vi "AixplorerArbitraryLoad.vi"() -> ()   [LabVIEW 2015]
uses:
  Tek shared libraries/ArbitraryFunctions/VImode.vi
  General Libraries/Sequences.lvlib
  Tek shared libraries/ArbitraryFunctions.lvlib
  Read and Save Files/RW_Protocols.lvlib
panel:
  in  "CH2":bool
  in  "CH1":bool
  in  "event trig":bool
  in  "run":bool
  in  "WaveDuration (us)":dbl=2e-05
  out "sample rate (Hz) 2":dbl
  in  "Freq US (Hz)":dbl=6000000.0
  in  "?":T1(tab)
  in  "Sequence Loop Initialization":T2(array[cluster])=[{"min"=0.0, "step"=0.25, "max"=1.0, "name"="Phase"}, {"min"=1.0, "step"=1.0, "max"=3.0, "name"="Harmonic"}]
  in  "manual sequence":bool
  in  "load data log":bool
  in  "Multicolumn Listbox":i32[](listbox)
  out "Waveform Graph":dbl[][](graph)
  in  "FileName":string="LogFile.csv"
  in  "Enum":enum16{"sinus", "triangle"}(ring)=enum."triangle"
  in  "N average":i32=500
  out "Freq CH2 (Hz)":dbl=100000.0
  in  "clear waveforms":bool
  in  "define waveform CH1":bool
  out "Low Frequency OUT":dbl=100000.0
  out "High Frequency OUT":dbl=100000.0
  out "error out":errorcluster
  in  "load sequence CH1":bool
  in  "channel":enum16{"CH1", "CH2"}(ring)=enum."CH2"
  in  "CH1 (VOLT)":dbl=0.5
  out "capabilities":T3
  in  "sequence repeat":i32=500
  in  "sample rate (Hz)":dbl
  in  "define waveform CH 2":bool
  in  "other button":bool
  in  "Stop Button":bool
  in  "resource name":refnum<k15>
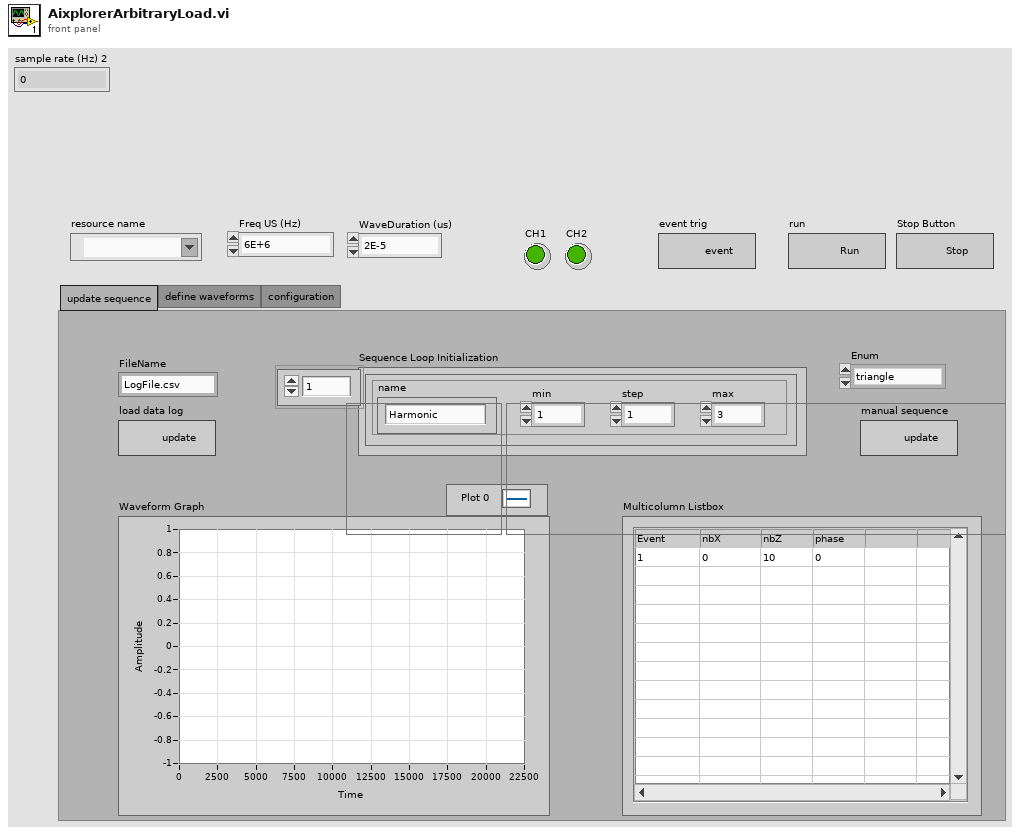
[diagram p1: front panel]
types:
  T1 = enum32{"update sequence", "define waveforms", "configuration"}
  T2 = cluster{"min":dbl, "step":dbl, "max":dbl, "name":string}[]
  T3 = cluster{"Max Number Of Sequences":i32, "Min Sequence Length":i32, "Max Sequence Length":i32, "Max Loop Count":i32}
  T4 = enum8{"Enabled", "Disabled", "Disabled and Grayed Out"}
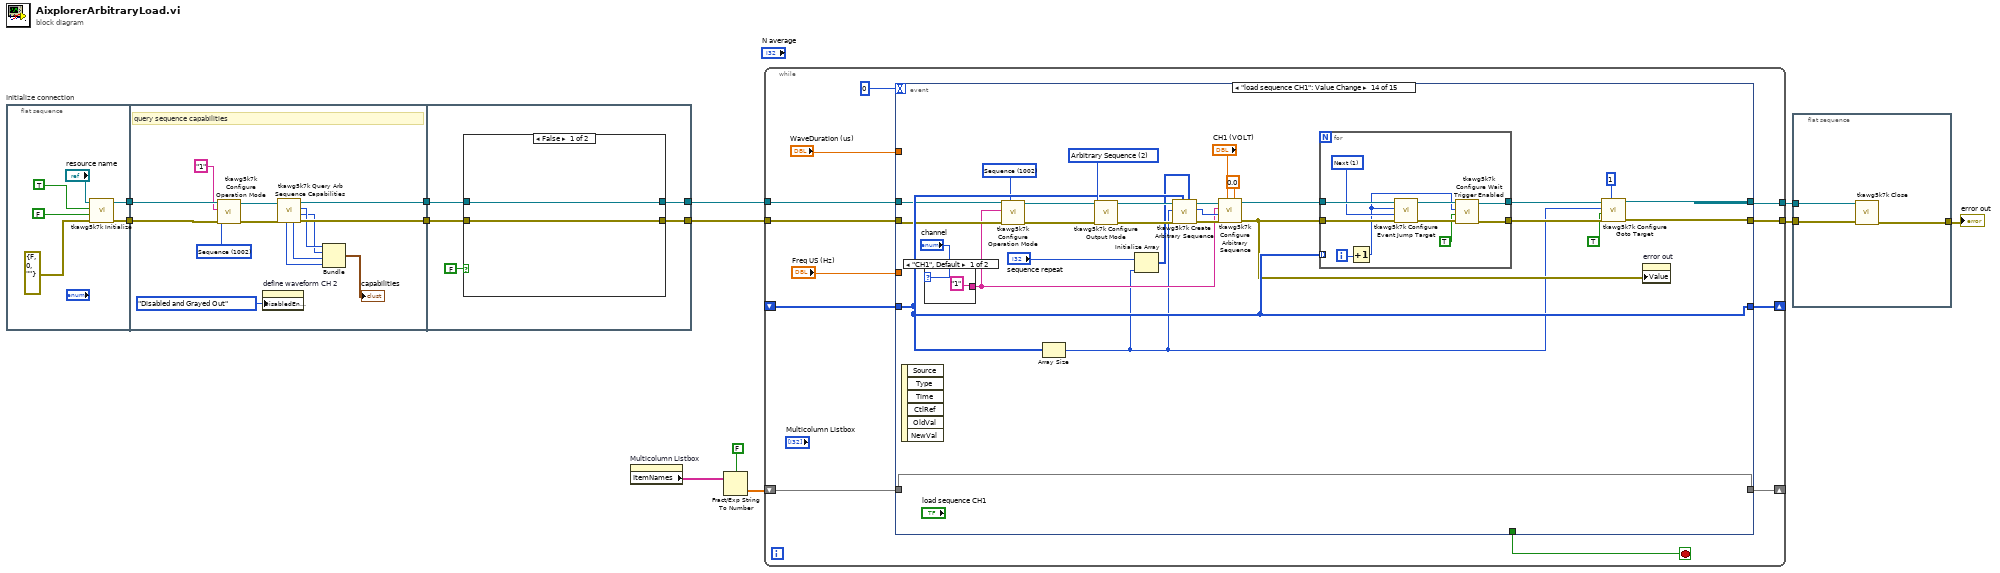
[diagram p0: block diagram]
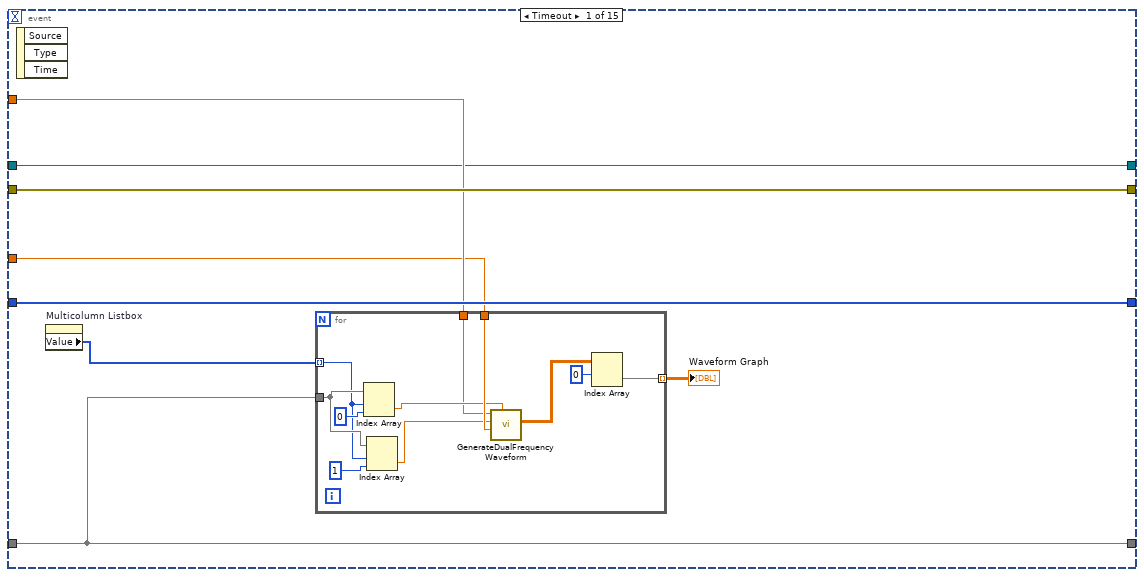
[diagram p2: hidden frame]
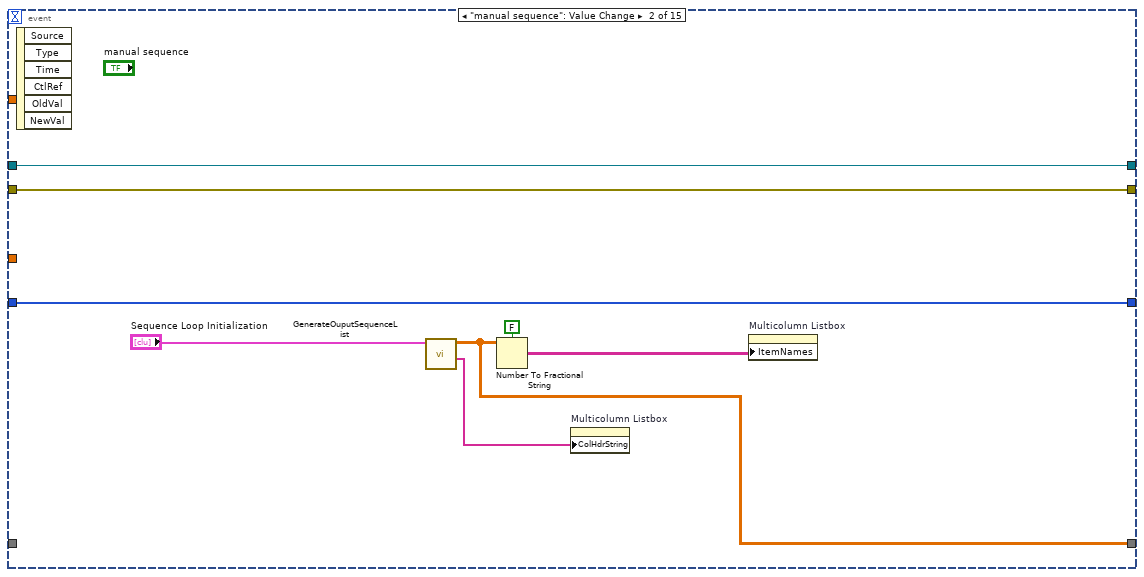
[diagram p3: hidden frame]
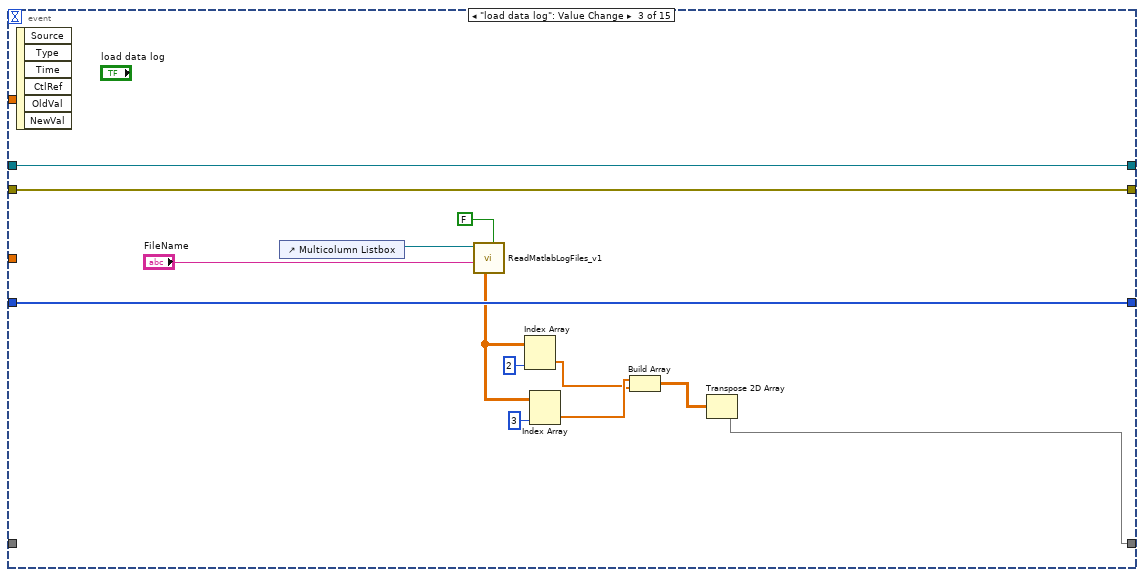
[diagram p4: hidden frame]
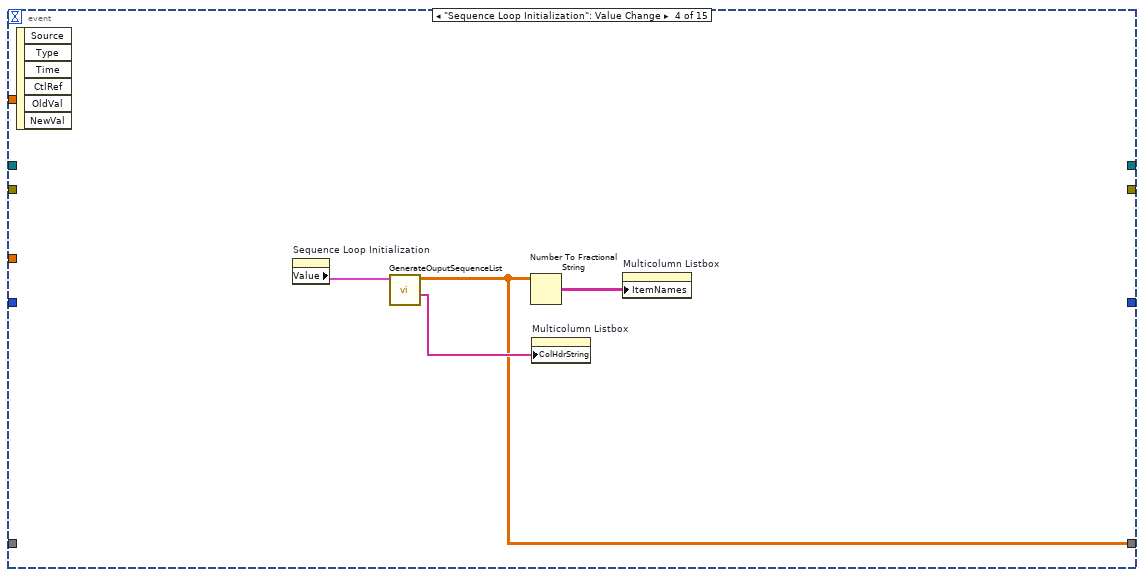
[diagram p5: hidden frame]
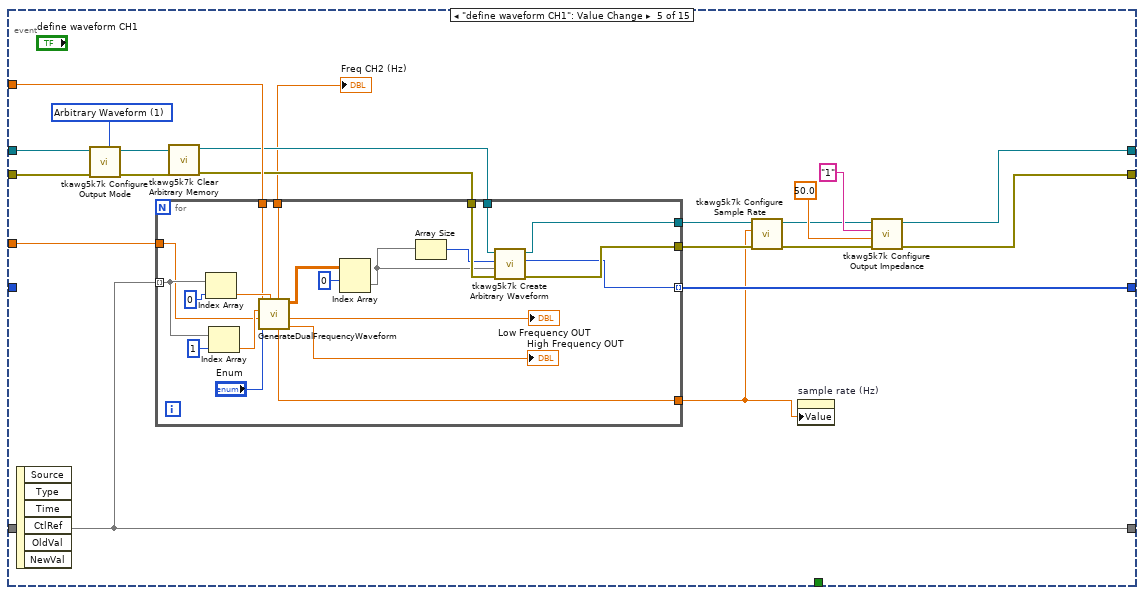
[diagram p6: hidden frame]
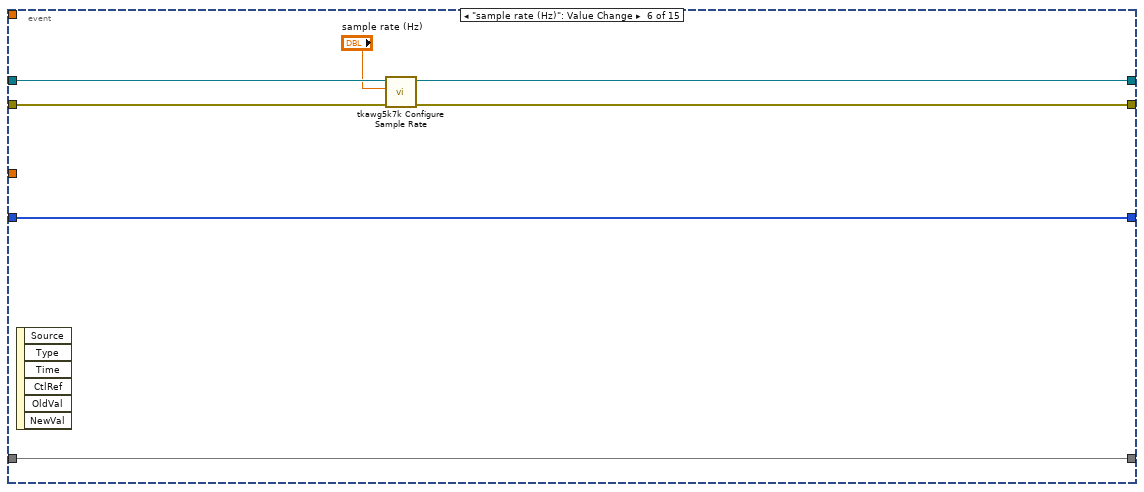
[diagram p7: hidden frame]
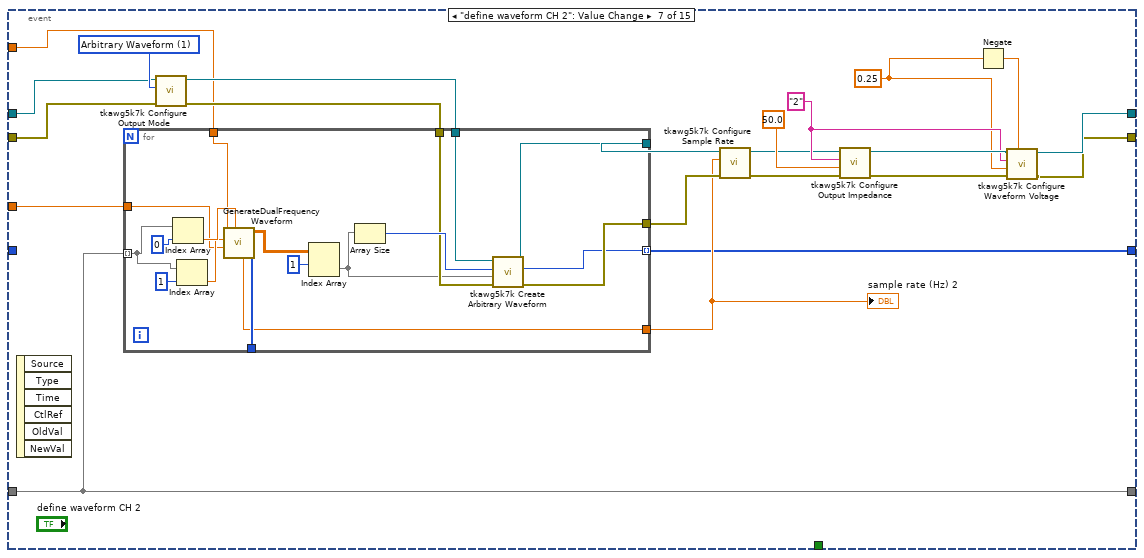
[diagram p8: hidden frame]
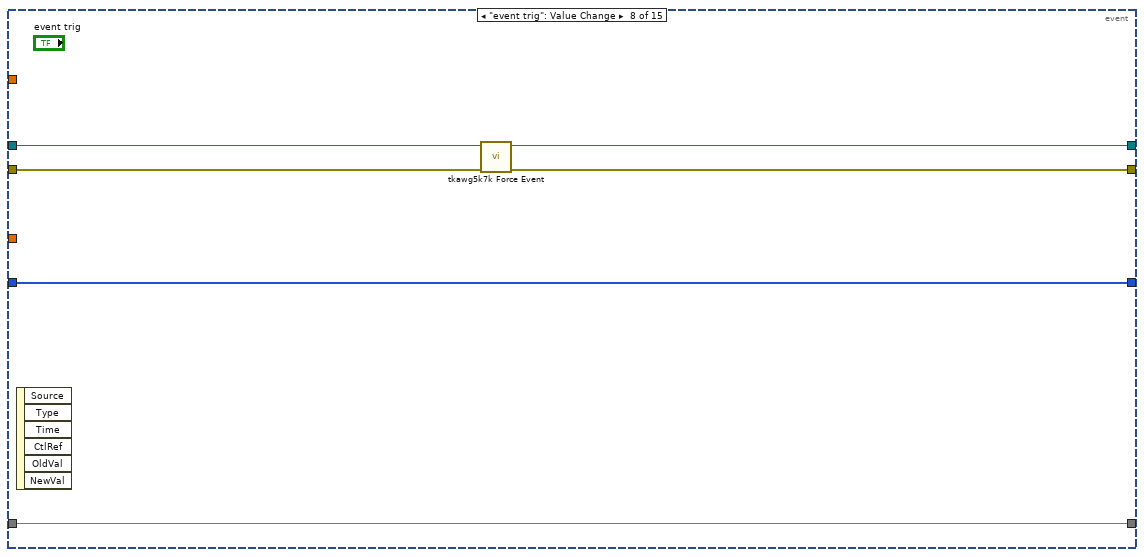
[diagram p9: hidden frame]
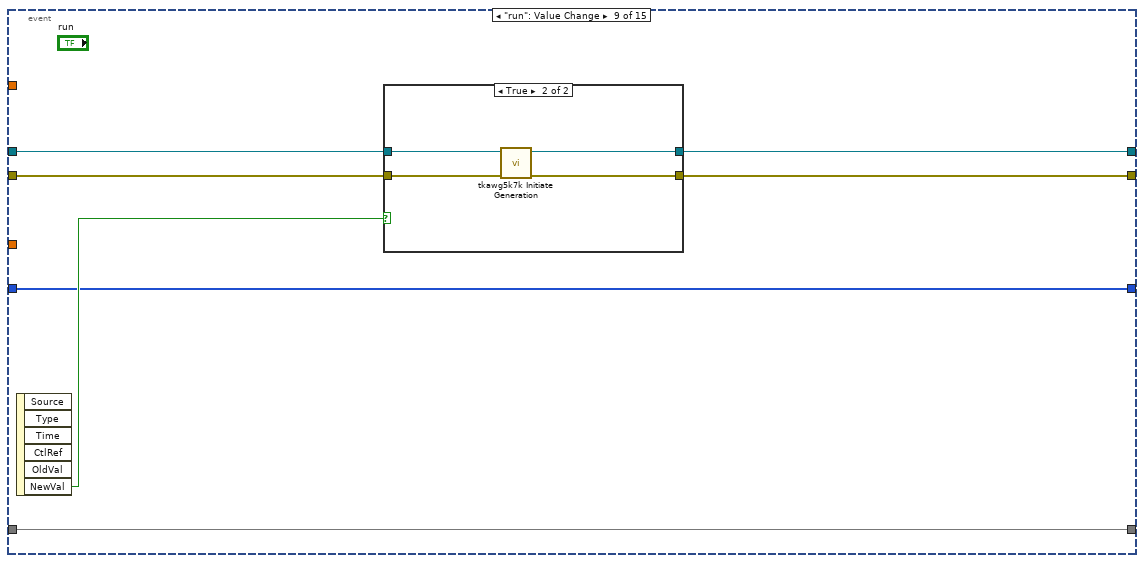
[diagram p10: hidden frame]
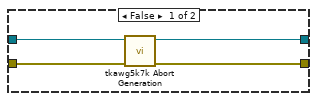
[diagram p11: hidden frame]
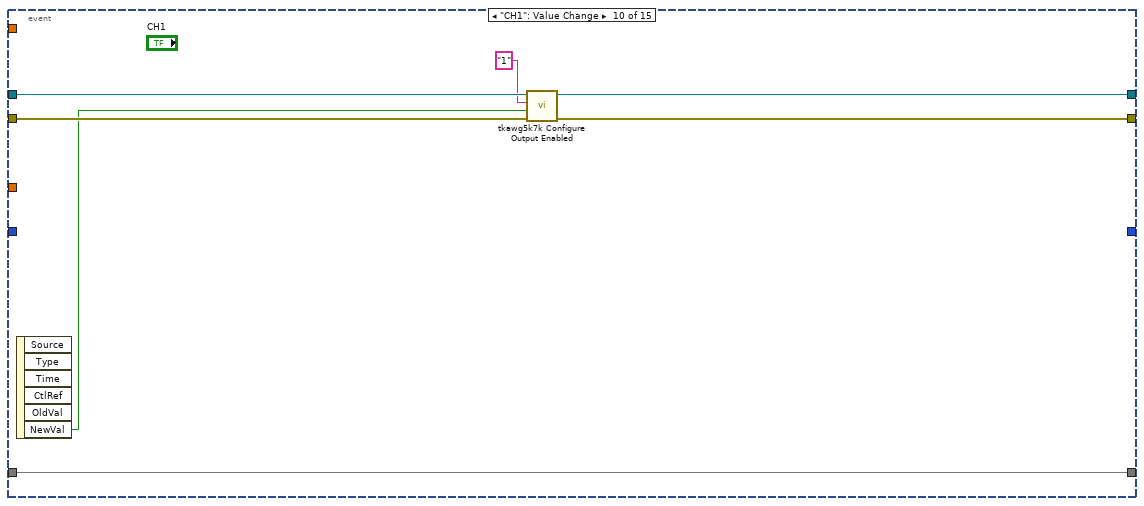
[diagram p12: hidden frame]
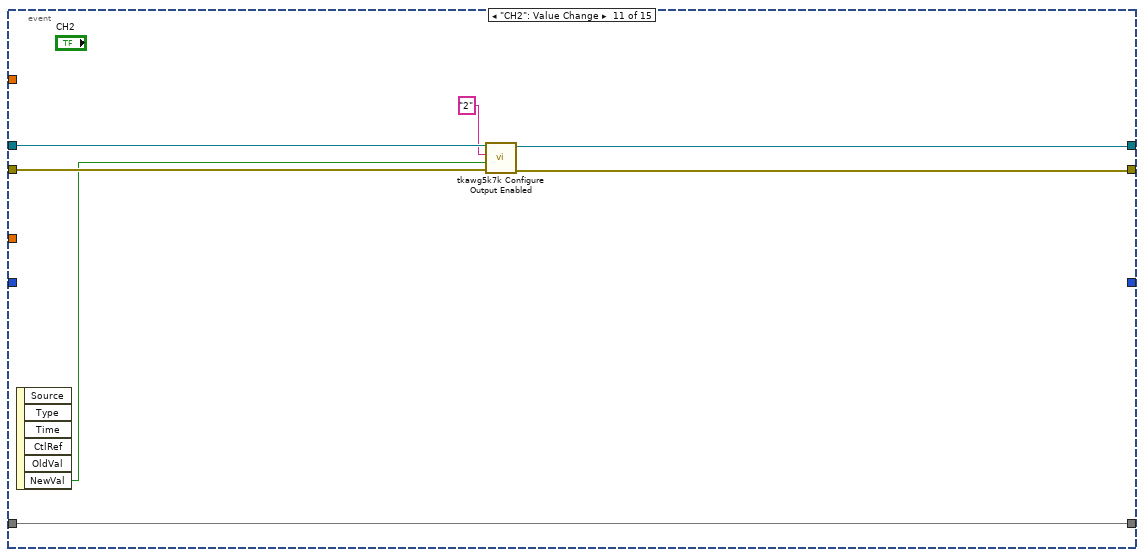
[diagram p13: hidden frame]
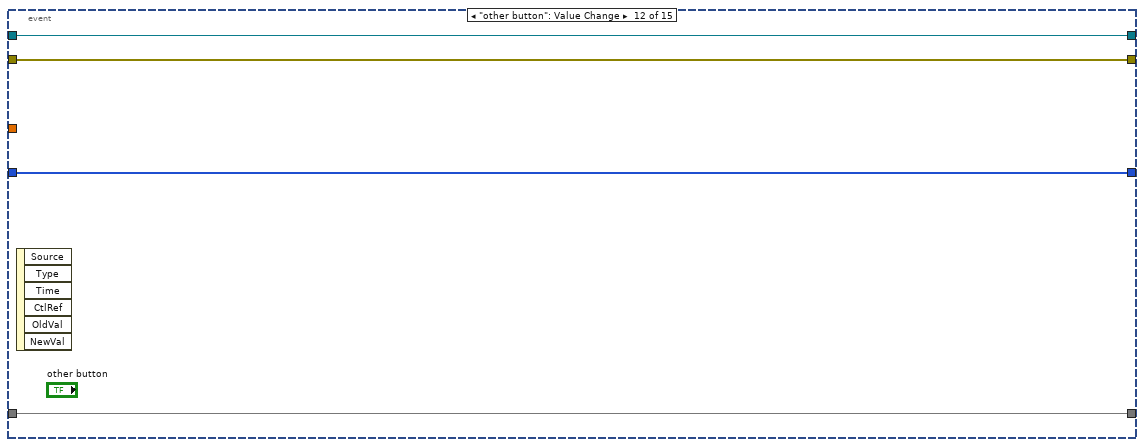
[diagram p14: hidden frame]
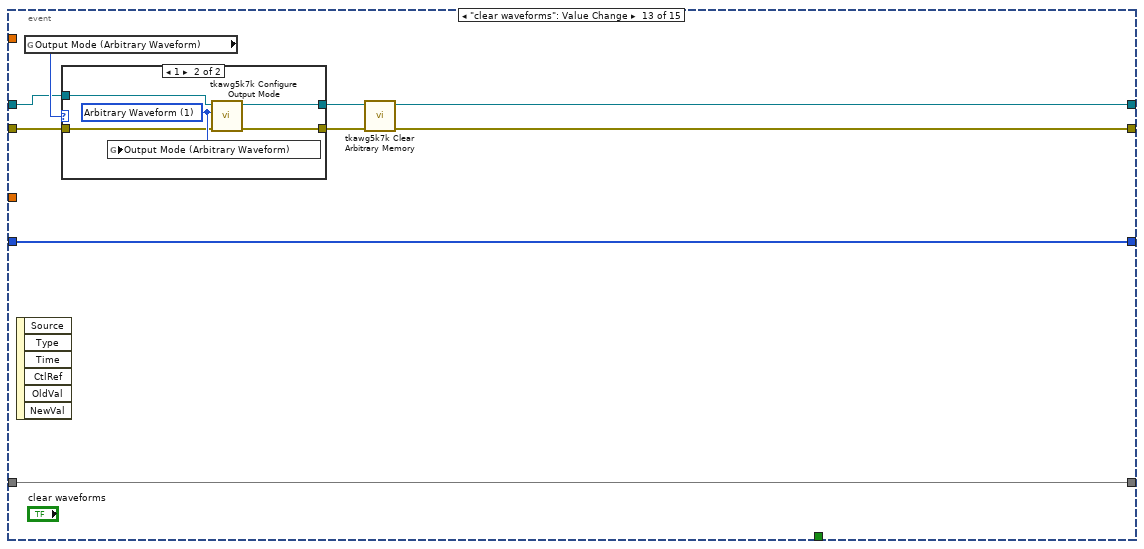
[diagram p15: hidden frame]
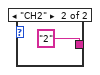
[diagram p17: hidden frame]
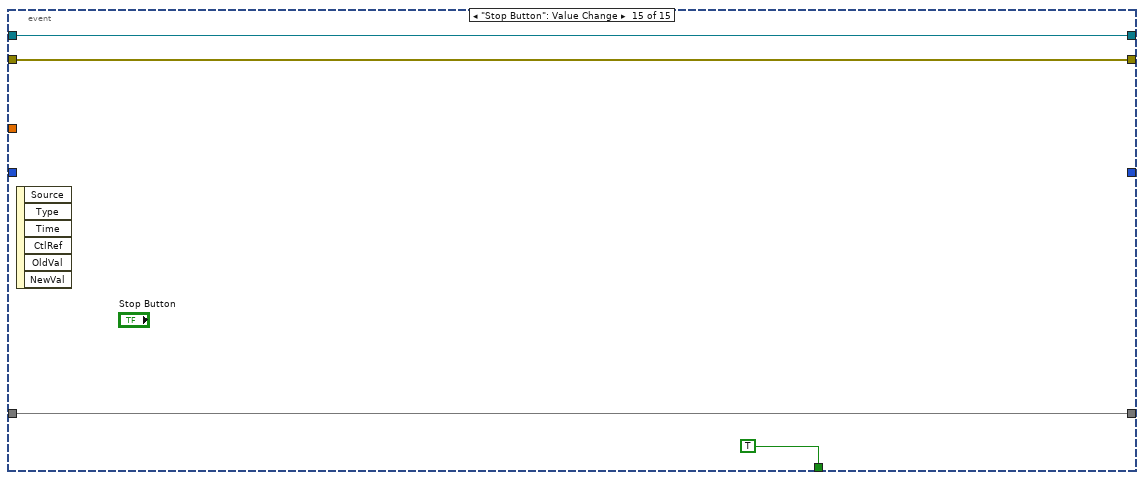
[diagram p18: hidden frame]
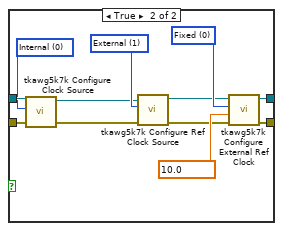
[diagram p19: hidden frame]
diagram:
  n1 = flat-sequence "Initialize connection" {
    tunnel: [w14] -> w4
    tunnel: [w13] -> w3
    tunnel: w4 -> [w31]
    tunnel: w3 -> [w32]
    tunnel: [w29] -> w2
    tunnel: [w27] -> w1
    tunnel: [w36] -> w11
    tunnel: [w37] -> w12
    tunnel: w2 -> [w35]
    tunnel: w1 -> [w34]
    frame #0 {
      n2 = call <instrlib>:"tkawg5k7k Initialize.vi"("error in (no error)"=errorcluster {"status"=FALSE, "code"=0, "source"=""}, "Reset Device (Yes)"=FALSE, "ID Query (Yes)"=TRUE, "resource name"="resource name") -> ("error out"=w13:errorcluster, "instrument handle out"=w14:refnum<k15>)  [unwired: 6 in]
    }
    frame #1 {
      w25 = 1002 items=["Continuous"=0, "Burst"=1, "Gated"=1001, "Sequence"=1002] ("Operation Mode (Continuous)")
      # "query sequence capabilities"
      n3 = call <instrlib>:"tkawg5k7k Configure Operation Mode.vi"("error in (no error)"=w32, "Operation Mode (Continuous)"=w25, "Channel Name (\"1\")"="1" ("Channel Name (\"1\")"), "instrument handle"=w31) -> ("error out"=w28:errorcluster, "instrument handle out"=w30:refnum<k15>)  [unwired: 6 in]
      n4 = property on="define waveform CH 2" class="Bool"("DisabledEnum"=T4."Disabled and Grayed Out" ("Disabled")) -> ()  [unwired: 2 in, 2 out]
      n5 = call <instrlib>:"tkawg5k7k Query Arb Sequence Capabilities.vi"("error in (no error)"=w28, "instrument handle"=w30) -> ("error out"=w27:errorcluster, "Min Sequence Length"=w23:i32, "Max Number Of Sequences"=w24:i32, "instrument handle out"=w29:refnum<k15>, "Max Sequence Length"=w22:i32, "Max Loop Count"=w21:i32)  [unwired: 4 in]
      n6 = Bundle("Max Number Of Sequences"=w24, "Min Sequence Length"=w23, "Max Sequence Length"=w22, "Max Loop Count"=w21) -> (→"capabilities":T3)  [unwired: 1 in]
    }
    frame #2 {
      n7 = case shown="False" FALSE {
        tunnel: [w39 w51] -> w37
        tunnel: [w38 w50] -> w36
        tunnel: w35 -> [w39 w44]
        tunnel: w34 -> [w38 w41]
        frame False {
        }
        frame True {
          w43 = 0 items=["Internal", "External", "External fixed", "External variable"] ("Clock Source (Internal)")
          w47 = 1 items=["Internal", "External"] ("Reference Clock Source (Internal)")
          w48 = 0 items=["Fixed", "Variable"] ("External Ref Type (Fixed)")
          w49 = 10.0 items=["10 MHz"=10.0, "20 MHz"=20.0, "100 MHz"=100.0] ("Ref Frequency (10 MHz)")
          n8 = call <instrlib>:"tkawg5k7k Configure Clock Source.vi"("error in (no error)"=w41, "Clock Source (Internal)"=w43, "instrument handle"=w44) -> ("error out"=w40:errorcluster, "instrument handle out"=w42:refnum<k15>)  [unwired: 7 in]
          n9 = call <instrlib>:"tkawg5k7k Configure Ref Clock Source.vi"("error in (no error)"=w40, "Reference Clock Source (Internal)"=w47, "instrument handle"=w42) -> ("error out"=w45:errorcluster, "instrument handle out"=w46:refnum<k15>)  [unwired: 7 in]
          n10 = call <instrlib>:"tkawg5k7k Configure External Ref Clock.vi"("error in (no error)"=w45, "Ref Frequency (10 MHz)"=w49, "External Ref Type (Fixed)"=w48, "instrument handle"=w46) -> ("error out"=w50:errorcluster, "instrument handle out"=w51:refnum<k15>)  [unwired: 6 in]
        }
      }
    }
  }
  n11 = property on="Multicolumn Listbox" class="MCListbox (strict)"() -> ("ItemNames"=w7:string[][])  [unwired: 2 in, 2 out]
  n12 = Fract/Exp String To Number(use system decimal point (T)=FALSE, string=w7) -> (number=w6:dbl[][])  [unwired: 2 in, 1 out]
  n13 = while {
    tunnel: w12 -> [w62]
    tunnel: w11 -> [w61]
    tunnel: [w63] -> w10
    tunnel: [w60] -> w9
    shift-right: [w57] -> _
    shift-left: w6 -> [w56]
    shift-right: [w55] -> _
    shift-left: _ -> [w54]
    stop <- w58 stop-if-true
    n14 = event shown="[13] \"load sequence CH1\": Value Change" {
      selector: _ -> [_ _ _ _ _ _ _ _ _ _ _ _ _ _ _]
      dyn-events: _ -> [_ _ _ _ _ _ _ _ _ _ _ _ _ _ _]
      timeout: 0 -> [_ _ _ _ _ _ _ _ _ _ _ _ _ _ _]
      tunnel: [w64 w86 w102 _ w116 w154 w162 w200 w204 w222 w229 w234 w237 w257 w293] -> w63
      tunnel: w62 -> [w64 w86 w102 _ w114 w156 w160 w202 w206 w224 w231 w234 w243 w264 w293]
      tunnel: w61 -> [w71 w85 w101 _ w113 w155 w159 w201 w205 w223 w230 w233 w242 w265 w294]
      tunnel: [w71 w85 w101 _ w115 w153 w161 w199 w203 w221 w228 w233 w239 w255 w294] -> w60
      tunnel: [_ _ _ _ _ _ _ _ _ _ _ _ _ _ TRUE] -> w58
      tunnel: [w66 w83 w91 w104 w128 w150 w157 w197 w207 w218 w225 w235 w236 w279 w292] -> w57
      tunnel: w56 -> [w66 _ _ _ w128 w150 w157 w197 w207 w218 w225 w235 w236 w279 w292]
      tunnel: [w70 w87 w103 _ w126 w152 w158 w198 w208 _ _ w232 w241 w274 _] -> w55
      tunnel: w54 -> [w70 w87 w103 _ _ w152 _ w198 w208 _ _ w232 w241 w274 _]
      tunnel: "WaveDuration (us)" -> [w69 _ _ _ w121 _ w163 _ _ _ _ _ _ _ _]
      tunnel: "Freq US (Hz)" -> [w68 _ _ _ w120 _ w164 _ _ _ _ _ _ _ _]
      event Timeout {
        n15 = event-data() -> ()  [unwired: 1 in, 3 out]
        n16 = property on="Multicolumn Listbox" class="MCListbox (strict)"() -> ("Value"=w67:i32[])  [unwired: 2 in, 2 out]
        n17 = for {
          tunnel: w69 -> [w75]
          tunnel: w68 -> [w82]
          tunnel: w67 -> [w76] mode=indexing
          tunnel: w66 -> [w81]
          tunnel: [w72] -> w65 mode=indexing
          n18 = Index Array(array=w81, index (row)=w76, index (col)=0 ("index")) -> (element=w77:dbl)
          n19 = Index Array(array=w81, index (row)=w76, index (col)=1 ("index")) -> (element=w78:dbl)
          n20 = call "GenerateDualFrequencyWaveform.vi"("Phase (2pi unit)"=w77, "Freq US (Hz)"=w82, "Harmonic"=w78, "WaveDuration (us)"=w75) -> ("Waveforms"=w74:dbl[][])  [unwired: 2 in, 5 out]
          n21 = Index Array(array=w74, index (row)=0) -> (element=w72:dbl[])  [unwired: 1 in]
        }
        "Waveform Graph" <- w65
      }
      event "manual sequence": Value Change {
        n22 = event-data() -> ()  [unwired: 1 in, 6 out]
        n23 = call "GenerateOuputSequenceList.vi"("input parameters"="Sequence Loop Initialization") -> ("output Names"=w89:string[], "output array"=w83:dbl[][])  [unwired: 9 in]
        n24 = Number To Fractional String(use system decimal point (T)=FALSE, number=w83) -> (F-format string=w88:string[][])  [unwired: 2 in]
        n25 = property on="Multicolumn Listbox" class="MCListbox (strict)"("ColHdrString"=w89) -> ()  [unwired: 2 in, 2 out]
        n26 = property on="Multicolumn Listbox" class="MCListbox (strict)"("ItemNames"=w88) -> ()  [unwired: 2 in, 2 out]
      }
      event "load data log": Value Change {
        n27 = event-data() -> ()  [unwired: 1 in, 6 out]
        n28 = control-ref of="Multicolumn Listbox"() -> (w100:refnum<vi>)
        n29 = call "ReadMatlabLogFiles_v1.vi"("use system decimal point (T)"=FALSE, "FileName"="FileName", "sequence list REF"=w100) -> ("all values"=w96:dbl[][])  [unwired: 4 in, 4 out]
        n30 = Index Array(array=w96, index (col)=2 ("disabled index (col)")) -> (element=w93:dbl[])  [unwired: 1 in]
        n31 = Index Array(array=w96, index (col)=3 ("disabled index (col)")) -> (element=w94:dbl[])  [unwired: 1 in]
        n32 = Build Array(w94, w93) -> (w92:dbl[][])
        n33 = Transpose 2D Array(2D array=w92) -> (transposed array=w91:dbl[][])
      }
      event "Sequence Loop Initialization": Value Change {
        n34 = event-data() -> ()  [unwired: 1 in, 6 out]
        n35 = property on="Sequence Loop Initialization" class="Arr (strict)"() -> ("Value"=w107:T2)  [unwired: 2 in, 2 out]
        n36 = call "GenerateOuputSequenceList.vi"("input parameters"=w107) -> ("output Names"=w105:string[], "output array"=w104:dbl[][])  [unwired: 9 in]
        n37 = Number To Fractional String(number=w104) -> (F-format string=w106:string[][])  [unwired: 3 in]
        n38 = property on="Multicolumn Listbox" class="MCListbox (strict)"("ColHdrString"=w105) -> ()  [unwired: 2 in, 2 out]
        n39 = property on="Multicolumn Listbox" class="MCListbox (strict)"("ItemNames"=w106) -> ()  [unwired: 2 in, 2 out]
      }
      event "define waveform CH1": Value Change {
        w127 = 1 items=["Arbitrary Waveform"=1, "Arbitrary Sequence"=2] ("Output Mode (Arbitrary Waveform)")
        n40 = event-data() -> ()  [unwired: 1 in, 6 out]
        n41 = call <instrlib>:"tkawg5k7k Configure Output Mode.vi"("error in (no error)"=w113, "Output Mode (Arbitrary Waveform)"=w127, "instrument handle"=w114) -> ("error out"=w112:errorcluster, "instrument handle out"=w110:refnum<k15>)  [unwired: 7 in]
        n42 = call <instrlib>:"tkawg5k7k Clear Arbitrary Memory.vi"("error in (no error)"=w112, "instrument handle"=w110) -> ("error out"=w111:errorcluster, "instrument handle out"=w109:refnum<k15>)  [unwired: 8 in]
        n43 = for {
          tunnel: w128 -> [w146] mode=indexing
          tunnel: w109 -> [w145]
          tunnel: w111 -> [w144]
          tunnel: [w130] -> w126 mode=indexing
          tunnel: w121 -> [w135]
          tunnel: [w143] -> w117
          tunnel: w120 -> [w131]
          tunnel: [w139] -> w119
          tunnel: [w138] -> w118
          tunnel: [w134] -> w108
          n44 = Index Array(array=w146, index=0) -> (element=w147:dbl)
          n45 = Index Array(array=w146, index=1) -> (element=w132:dbl)
          n46 = call "GenerateDualFrequencyWaveform.vi"("Phase (2pi unit)"=w147, "Enum"="Enum", "Freq US (Hz)"=w131, "Harmonic"=w132, "WaveDuration (us)"=w135) -> ("High Frequency OUT"=→"High Frequency OUT":dbl, "Low Frequency OUT"=→"Low Frequency OUT":dbl, "Waveforms"=w141:dbl[][], "Sample Frequency (Hz)"=w143:dbl, "Freq CH2 (Hz)"=w134:dbl)  [unwired: 1 in, 1 out]
          n47 = Index Array(array=w141, index (row)=0) -> (element=w133:dbl[])  [unwired: 1 in]
          n48 = Array Size(array=w133) -> (size(s)=w140:i32)
          n49 = call <instrlib>:"tkawg5k7k Create Arbitrary Waveform.vi"("error in (no error)"=w144, "Waveform Data Array"=w133, "Waveform Size"=w140, "instrument handle"=w145) -> ("error out"=w138:errorcluster, "Waveform Handle"=w130:i32, "instrument handle out"=w139:refnum<k15>)  [unwired: 5 in]
        }
        "Freq CH2 (Hz)" <- w108
        n50 = call <instrlib>:"tkawg5k7k Configure Sample Rate.vi"("error in (no error)"=w118, "Sample Rate (5.0e+8)"=w117, "instrument handle"=w119) -> ("error out"=w123:errorcluster, "instrument handle out"=w122:refnum<k15>)  [unwired: 7 in]
        n51 = property on="sample rate (Hz)" class="DigNum (strict)"("Value"=w117) -> ()  [unwired: 2 in, 2 out]
        n52 = call <instrlib>:"tkawg5k7k Configure Output Impedance.vi"("error in (no error)"=w123, "Impedance (50.0)"=50.0, "Channel Name (\"1\")"="1" ("Channel Name (\"1\")"), "instrument handle"=w122) -> ("error out"=w115:errorcluster, "instrument handle out"=w116:refnum<k15>)  [unwired: 6 in]
      }
      event "sample rate (Hz)": Value Change {
        n53 = event-data() -> ()  [unwired: 1 in, 6 out]
        n54 = call <instrlib>:"tkawg5k7k Configure Sample Rate.vi"("error in (no error)"=w155, "Sample Rate (5.0e+8)"="sample rate (Hz)", "instrument handle"=w156) -> ("error out"=w153:errorcluster, "instrument handle out"=w154:refnum<k15>)  [unwired: 7 in]
      }
      event "define waveform CH 2": Value Change {
        w166 = 0.25 ("High Voltage (0.25)")
        w173 = "2" ("Channel Name (\"1\")")
        w176 = 1 items=["Arbitrary Waveform"=1, "Arbitrary Sequence"=2] ("Output Mode (Arbitrary Waveform)")
        n55 = event-data() -> ()  [unwired: 1 in, 6 out]
        n56 = call <instrlib>:"tkawg5k7k Configure Output Mode.vi"("error in (no error)"=w159, "Output Mode (Arbitrary Waveform)"=w176, "instrument handle"=w160) -> ("error out"=w178:errorcluster, "instrument handle out"=w177:refnum<k15>)  [unwired: 7 in]
        n57 = for {
          tunnel: w177 -> [w182]
          tunnel: w178 -> [w181]
          tunnel: [w190] -> w170
          tunnel: [w188] -> w171
          tunnel: [w194] -> _
          tunnel: [w193] -> w167
          tunnel: [w189] -> w158 mode=indexing
          tunnel: w164 -> [w183]
          tunnel: w157 -> [w186] mode=indexing
          tunnel: w163 -> [w180]
          n58 = Index Array(array=w186, index=0) -> (element=w185:dbl)
          n59 = Index Array(array=w186, index=1) -> (element=w184:dbl)
          n60 = call "GenerateDualFrequencyWaveform.vi"("Phase (2pi unit)"=w185, "Freq US (Hz)"=w183, "Harmonic"=w184, "WaveDuration (us)"=w180) -> ("Waveforms"=w192:dbl[][], "OutPut Points"=w194:i32[], "Sample Frequency (Hz)"=w193:dbl)  [unwired: 2 in, 3 out]
          n61 = Index Array(array=w192, index (row)=1) -> (element=w179:dbl[])  [unwired: 1 in]
          n62 = Array Size(array=w179) -> (size(s)=w187:i32)
          n63 = call <instrlib>:"tkawg5k7k Create Arbitrary Waveform.vi"("error in (no error)"=w181, "Waveform Data Array"=w179, "Waveform Size"=w187, "instrument handle"=w182) -> ("error out"=w190:errorcluster, "Waveform Handle"=w189:i32, "instrument handle out"=w188:refnum<k15>)  [unwired: 5 in]
        }
        "sample rate (Hz) 2" <- w167
        n64 = call <instrlib>:"tkawg5k7k Configure Sample Rate.vi"("error in (no error)"=w170, "Sample Rate (5.0e+8)"=w167, "instrument handle"=w171) -> ("error out"=w169:errorcluster, "instrument handle out"=w168:refnum<k15>)  [unwired: 7 in]
        n65 = call <instrlib>:"tkawg5k7k Configure Output Impedance.vi"("error in (no error)"=w169, "Impedance (50.0)"=50.0, "Channel Name (\"1\")"=w173, "instrument handle"=w168) -> ("error out"=w172:errorcluster, "instrument handle out"=w174:refnum<k15>)  [unwired: 6 in]
        n66 = Negate(x=w166) -> (-x=w165:dbl)
        n67 = call <instrlib>:"tkawg5k7k Configure Waveform Voltage.vi"("Low Voltage (-0.25)"=w165, "error in (no error)"=w172, "High Voltage (0.25)"=w166, "Channel Name (\"1\")"=w173, "instrument handle"=w174) -> ("error out"=w161:errorcluster, "instrument handle out"=w162:refnum<k15>)  [unwired: 5 in]
      }
      event "event trig": Value Change {
        n68 = event-data() -> ()  [unwired: 1 in, 6 out]
        n69 = call <instrlib>:"tkawg5k7k Force Event.vi"("error in (no error)"=w201, "instrument handle"=w202) -> ("error out"=w199:errorcluster, "instrument handle out"=w200:refnum<k15>)  [unwired: 8 in]
      }
      event "run": Value Change {
        n70 = event-data() -> ("NewVal"=w209:bool)  [unwired: 1 in, 5 out]
        n71 = case shown="True" w209 {
          tunnel: w206 -> [w213 w217]
          tunnel: w205 -> [w212 w215]
          tunnel: [w211 w216] -> w204
          tunnel: [w210 w214] -> w203
          frame False {
            n72 = call <instrlib>:"tkawg5k7k Abort Generation.vi"("error in (no error)"=w212, "instrument handle"=w213) -> ("error out"=w210:errorcluster, "instrument handle out"=w211:refnum<k15>)  [unwired: 8 in]
          }
          frame True {
            n73 = call <instrlib>:"tkawg5k7k Initiate Generation.vi"("error in (no error)"=w215, "instrument handle"=w217) -> ("error out"=w214:errorcluster, "instrument handle out"=w216:refnum<k15>)  [unwired: 8 in]
          }
        }
      }
      event "CH1": Value Change {
        n74 = event-data() -> ("NewVal"=w219:bool)  [unwired: 1 in, 5 out]
        n75 = call <instrlib>:"tkawg5k7k Configure Output Enabled.vi"("error in (no error)"=w223, "Channel Enabled (True)"=w219, "Channel Name (\"1\")"="1" ("Channel Name (\"1\")"), "instrument handle"=w224) -> ("error out"=w221:errorcluster, "instrument handle out"=w222:refnum<k15>)  [unwired: 6 in]
      }
      event "CH2": Value Change {
        n76 = event-data() -> ("NewVal"=w227:bool)  [unwired: 1 in, 5 out]
        n77 = call <instrlib>:"tkawg5k7k Configure Output Enabled.vi"("error in (no error)"=w230, "Channel Enabled (True)"=w227, "Channel Name (\"1\")"="2" ("Channel Name (\"1\")"), "instrument handle"=w231) -> ("error out"=w228:errorcluster, "instrument handle out"=w229:refnum<k15>)  [unwired: 6 in]
      }
      event "other button": Value Change {
        n78 = event-data() -> ()  [unwired: 1 in, 6 out]
      }
      event "clear waveforms": Value Change {
        n79 = event-data() -> ()  [unwired: 1 in, 6 out]
        n80 = global read "VImode.vi" "Output Mode (Arbitrary Waveform)"() -> (w244:i32)
        n81 = case shown="1" w244 {
          tunnel: w243 -> [w246 w250]
          tunnel: w242 -> [w245 w249]
          tunnel: [w246 w248] -> w238
          tunnel: [w245 w247] -> w240
          frame 0, Default {
          }
          frame 1 {
            w251 = 1 items=["Arbitrary Waveform"=1, "Arbitrary Sequence"=2] ("Output Mode (Arbitrary Waveform)")
            n82 = global write "VImode.vi" "Output Mode (Arbitrary Waveform)"(w251) -> ()
            n83 = call <instrlib>:"tkawg5k7k Configure Output Mode.vi"("error in (no error)"=w249, "Output Mode (Arbitrary Waveform)"=w251, "instrument handle"=w250) -> ("error out"=w247:errorcluster, "instrument handle out"=w248:refnum<k15>)  [unwired: 7 in]
          }
        }
        n84 = call <instrlib>:"tkawg5k7k Clear Arbitrary Memory.vi"("error in (no error)"=w240, "instrument handle"=w238) -> ("error out"=w239:errorcluster, "instrument handle out"=w237:refnum<k15>)  [unwired: 8 in]
      }
      event "load sequence CH1": Value Change {
        w266 = 1002 items=["Continuous"=0, "Burst"=1, "Gated"=1001, "Sequence"=1002] ("Operation Mode (Continuous)")
        w275 = 2 items=["Arbitrary Waveform"=1, "Arbitrary Sequence"=2] ("Output Mode (Arbitrary Waveform)")
        n85 = event-data() -> ()  [unwired: 1 in, 6 out]
        n86 = case shown="\"CH1\", Default" "channel" {
          tunnel: ["1" ("Channel Name (\"1\")") "2" ("Channel Name (\"1\")")] -> w263
          frame "CH1", Default {
          }
          frame "CH2" {
          }
        }
        n87 = call <instrlib>:"tkawg5k7k Configure Operation Mode.vi"("error in (no error)"=w265, "Operation Mode (Continuous)"=w266, "Channel Name (\"1\")"=w263, "instrument handle"=w264) -> ("error out"=w260:errorcluster, "instrument handle out"=w261:refnum<k15>)  [unwired: 6 in]
        n88 = Array Size(array=w274) -> (size(s)=w252:i32)
        n89 = call <instrlib>:"tkawg5k7k Configure Output Mode.vi"("error in (no error)"=w260, "Output Mode (Arbitrary Waveform)"=w275, "instrument handle"=w261) -> ("error out"=w276:errorcluster, "instrument handle out"=w277:refnum<k15>)  [unwired: 7 in]
        n90 = Initialize Array("sequence repeat", w252) -> (w270:i32[])
        n91 = call <instrlib>:"tkawg5k7k Create Arbitrary Sequence.vi"("Loop Counts Array"=w270, "Waveform Handles Array"=w274, "error in (no error)"=w276, "Sequence Length"=w252, "instrument handle"=w277) -> ("error out"=w271:errorcluster, "Sequence Handle"=w278:i32, "instrument handle out"=w272:refnum<k15>)  [unwired: 4 in]
        n92 = call <instrlib>:"tkawg5k7k Configure Arbitrary Sequence.vi"("Offset (0.00)"=0.0, "Gain (1.00)"="CH1 (VOLT)", "error in (no error)"=w271, "Sequence Handle"=w278, "Channel Name (\"1\")"=w263, "instrument handle"=w272) -> ("error out"=w262:errorcluster, "instrument handle out"=w273:refnum<k15>)  [unwired: 4 in]
        n93 = for {
          tunnel: w274 -> [_] mode=indexing
          tunnel: w262 -> [w290]
          tunnel: [w284] -> w256
          tunnel: w273 -> [w289]
          tunnel: [w286] -> w258
          i -> [w291]
          w288 = 1 items=["Index", "Next", "Off"] ("Jump Type (Off)")
          n94 = Increment(x=w291) -> (x+1=w283:i32)
          n95 = call <instrlib>:"tkawg5k7k Configure Event Jump Target.vi"("error in (no error)"=w290, "Jump Type (Off)"=w288, "Element (1)"=w283, "instrument handle"=w289) -> ("error out"=w285:errorcluster, "instrument handle out"=w287:refnum<k15>)  [unwired: 6 in]
          n96 = call <instrlib>:"tkawg5k7k Configure Wait Trigger Enabled.vi"("error in (no error)"=w285, "Enabled (False)"=TRUE, "Element (1)"=w283, "instrument handle"=w287) -> ("error out"=w284:errorcluster, "instrument handle out"=w286:refnum<k15>)  [unwired: 6 in]
        }
        n97 = call <instrlib>:"tkawg5k7k Configure Goto Target.vi"("Target Index (2)"=1, "error in (no error)"=w256, "Enabled (False)"=TRUE, "Element (1)"=w252, "instrument handle"=w258) -> ("error out"=w255:errorcluster, "instrument handle out"=w257:refnum<k15>)  [unwired: 5 in]
        n98 = property on="error out" class="Clust (strict)"("Value"=w262) -> ()  [unwired: 2 in, 2 out]
      }
      event "Stop Button": Value Change {
        n99 = event-data() -> ()  [unwired: 1 in, 6 out]
      }
    }
  }
  n100 = flat-sequence {
    tunnel: w10 -> [w296]
    tunnel: w9 -> [w298]
    tunnel: [w297] -> w8
    frame #0 {
      n101 = call <instrlib>:"tkawg5k7k Close.vi"("error in (no error)"=w298, "instrument handle"=w296) -> ("error out"=w297:errorcluster)  [unwired: 9 in]
    }
  }
  "error out" <- w8
